vi "Unreserve Sessions.vi"(8 "error in":errorcluster, 11 "session reservation in":refnum<class "Session Reservation.lvclass">) -> (0 "error out":errorcluster)   [LabVIEW 2020, in "Plug-In SDK Session Management V1.lvlib" / "Session Reservation.lvclass"]
doc: "Unreserves all sessions. Once this VI is called, the session reservation refnum is no longer valid."
uses:
  Session Reservation.lvclass
  Session Reservation.lvclass/Session Reservation.ctl
  gRPC/Generated APIs/ni/measurementlink/sessionmanagement/v1/RPC Messages/ni_measurementlink_sessionmanagement_v1_UnreserveSessionsRequest.ctl
  gRPC/Generated APIs/ni/measurementlink/sessionmanagement/v1/RPC Messages/ni_measurementlink_sessionmanagement_v1_SessionInformation.ctl
  gRPC/Generated APIs/ni/measurementlink/sessionmanagement/v1/RPC Messages/nidevice_grpc_Session.ctl
  gRPC/Generated APIs/ni/measurementlink/sessionmanagement/v1/RPC Messages/ni_measurementlink_sessionmanagement_v1_ChannelMapping.ctl
  Measurements/Helpers/Error Strings Global Internal.vi
  <vilib>/Utility/error.llb/Error Cluster From Error Code.vi
  IReservation Observer/IReservation Observer.lvclass
  gRPC/Generated APIs/ni/measurementlink/sessionmanagement/v1/ni.measurementlink.sessionmanagement.v1.lvlib
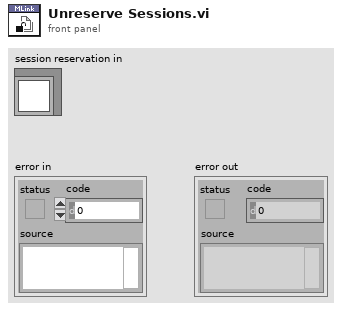
[diagram p1: front panel]
types:
  T1 = typedef "ni.measurementlink.sessionmanagement.v1.lvlib/ni_measurementlink_sessionmanagement_v1_UnreserveSessionsRequest.ctl" = cluster{"sessions":T2[]}
  T2 = typedef "ni.measurementlink.sessionmanagement.v1.lvlib/ni_measurementlink_sessionmanagement_v1_SessionInformation.ctl" = cluster{"session":T3, "resource_name":string, "channel_list":string, "instrument_type_id":string, "session_exists":bool, "channel_mappings":T4[]}
  T3 = typedef "ni.measurementlink.sessionmanagement.v1.lvlib/nidevice_grpc_Session.ctl" = cluster{"name":string}
  T4 = typedef "ni.measurementlink.sessionmanagement.v1.lvlib/ni_measurementlink_sessionmanagement_v1_ChannelMapping.ctl" = cluster{"pin_or_relay_name":string, "site":i32, "channel":string, "multiplexer_resource_name":string, "multiplexer_route":string}
  T5 = typedef "Plug-In SDK Session Management V1.lvlib/Session Reservation.lvclass/Data.ctl" = cluster{"session and driver infos":T6[], "pin or relay names":string[], "connection map":refnum<class "Connection Map.lvclass">, "pin map context":T8, "reservation observer":refnum<class "IReservation Observer.lvclass">, "dvr valid":bool, "group mappings":T9}
  T6 = typedef "Plug-In SDK Session Management V1.lvlib/Session Reservation.lvclass/Session and Driver Info.ctl" = cluster{"session info":T2, "session":variant, "session factory":refnum<class "ISession Factory.lvclass">, "initialize and close session behavior":T7}
  T7 = typedef "Instrument Sessions.lvlib/ISession Factory.lvclass/Initialize and Close Session Behavior.ctl" = enum16{"Initialize and Close", "Attach and Detach", "Initialize and Detach", "Attach and Close"}
  T8 = typedef "ni.measurementlink.sessionmanagement.v1.lvlib/ni_measurementlink_PinMapContext.ctl" = cluster{"pin_map_id":string, "sites":i32[]}
  T9 = typedef "Plug-In SDK Session Management V1.lvlib/Session Reservation.lvclass/Group Mapping.ctl" = map{string, string[]}
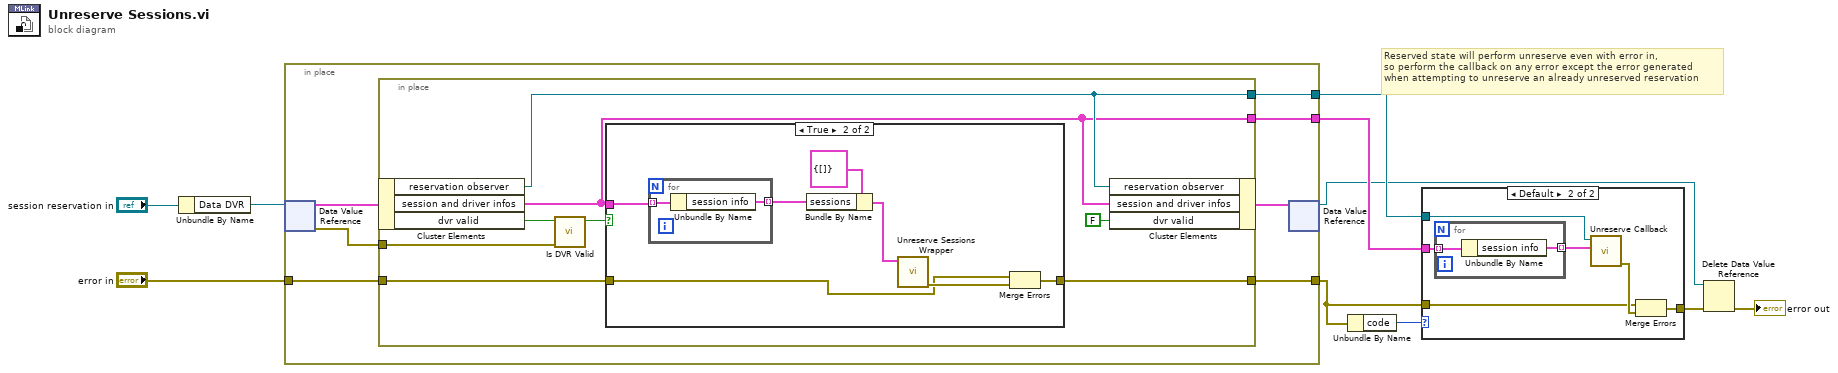
[diagram p0: block diagram]
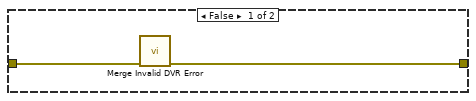
[diagram p2: hidden frame]
diagram:
  # "Reserved state will perform unreserve even with error in,\nso perform the callback on any error except the error generated\nwhen attempting to unreserve an already unreserved reservation"
  n1 = Unbundle By Name("session reservation in") -> ("Data DVR"=w8:refnum<data-value>)
  n2 = in-place {
    in-place-border: "error in" -> [w16]
    in-place-border: [w17] -> w4
    in-place-border: [w15] -> w7
    in-place-border: [w14] -> w5
    n3 = in-place-dvr #1(w8) -> (w13:T5, w11:errorcluster)
    n4 = in-place {
      in-place-border: [w18] -> w17
      in-place-border: w16 -> [w25]
      in-place-border: w11 -> [w24]
      in-place-border: [w20] -> w15
      in-place-border: [w19] -> w14
      n5 = in-place-cluster #2(w13) -> ("reservation observer"=w20:refnum<class "IReservation Observer.lvclass">, "session and driver infos"=w19:T6[], "dvr valid"=w22:bool)
      n6 = call "Is DVR Valid.vi"("dvr error in"=w24, "dvr valid in"=w22) -> ("dvr valid out"=w23:bool)  [unwired: 9 in]
      n7 = case shown="True" w23 {
        tunnel: w19 -> [_ w28]
        tunnel: [w26 w30] -> w18
        tunnel: w25 -> [w27 w29]
        frame False {
          n8 = call "Merge Invalid DVR Error.vi"("error in"=w27) -> ("error out"=w26:errorcluster)  [unwired: 10 in]
        }
        frame True {
          n9 = for {
            tunnel: w28 -> [w36] mode=indexing
            tunnel: [w35] -> w32 mode=indexing
            n10 = Unbundle By Name(w36) -> ("session info"=w35:T2)
          }
          n11 = Bundle By Name(cluster=T1 {"sessions"=[]} ("Request Data"), "sessions"=w32) -> (w31:T1)
          n12 = call "Unreserve Sessions Wrapper.vi"("request data"=w31) -> ("error out"=w34:errorcluster)  [unwired: 9 in, 1 out]
          n13 = Merge Errors(w29, w34) -> (w30:errorcluster)
        }
      }
      n14 = in-place-cluster #2("reservation observer"=w20, "session and driver infos"=w19, "dvr valid"=FALSE) -> (w12:T5)
    }
    n15 = in-place-dvr #1(w12) -> (w1:refnum<data-value>)  [unwired: 1 out]
  }
  n16 = Unbundle By Name(w4) -> ("code"=w6:i32)
  n17 = case shown="Default" w6 {
    tunnel: w4 -> [w37 w38]
    tunnel: [w37 w39] -> w3
    tunnel: w5 -> [_ w41]
    tunnel: w7 -> [_ w40]
    frame 5065 {
    }
    frame Default {
      n18 = for {
        tunnel: w41 -> [w45] mode=indexing
        tunnel: [w44] -> w43 mode=indexing
        n19 = Unbundle By Name(w45) -> ("session info"=w44:T2)
      }
      n20 = call-dynamic "Unreserve Callback.vi"("session infos"=w43, "reservation observer in"=w40) -> ("error out"=w42:errorcluster)  [unwired: 8 in, 1 out]
      n21 = Merge Errors(w38, w42) -> (w39:errorcluster)
    }
  }
  n22 = Delete Data Value Reference(data value reference=w1, error in=w3) -> (error out=→"error out":errorcluster)  [unwired: 1 out]
